vi "getDeviceType.vi"(8 "error in (no error)":errorcluster, 11 "DoDeviceData in":refnum<class "DoDeviceData.lvclass">) -> (0 "error out":errorcluster, 2 "type":T1(ring), 3 "DoDeviceData out":refnum<class "DoDeviceData.lvclass">)   [LabVIEW 2009, in "DataMappers.lvlib" / "DoDeviceData.lvclass"]
uses:
  DoDeviceData.lvclass
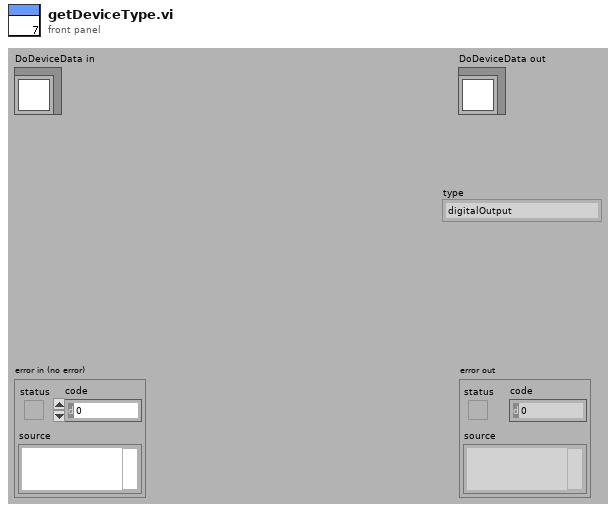
[diagram p1: front panel]
types:
  T1 = enum16{"digitalOutput", "digitalInput", "analogOutput", "analogInput", "rfOutput", "ethernetSupply"}
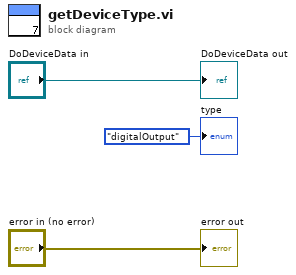
[diagram p0: block diagram]
diagram:
  "error out" <- "error in (no error)"
  "DoDeviceData out" <- "DoDeviceData in"
  "type" <- T1."digitalOutput" ("type")
